vi "Get Switch Heat.vi"(8 "error in (no error)":errorcluster, 11 "Instrument.1820 in":refnum<class "Instrument.Oxford1820.lvclass">) -> (0 "error out":errorcluster, 1 "Heater On?":bool, 2 "Switch Heater Status":string, 3 "Instrument.1820 in":refnum<class "Instrument.Oxford1820.lvclass">)   [LabVIEW 2016, in "Instrument.Oxford1820.lvclass"]
uses:
  Instrument.Oxford1820.lvclass
  Typedefs/Instrument.Oxford1820.Commands-enum.ctl
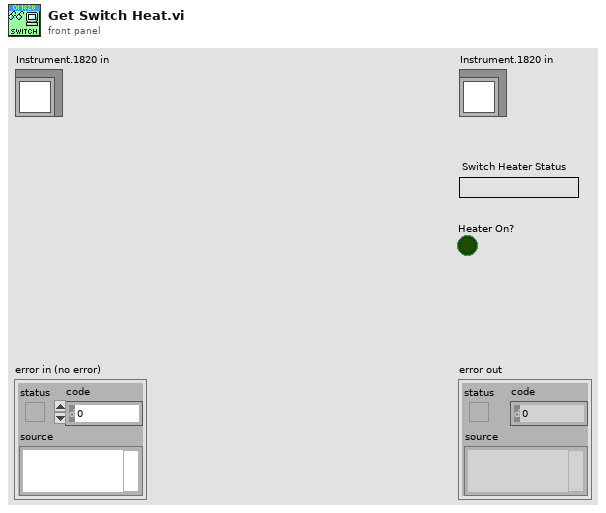
[diagram p1: front panel]
types:
  T1 = typedef "Instrument.Oxford1820.lvclass/Instrument.Oxford1820.Commands-enum.ctl" = enum16{"setAction", "setTarget", "setSwitchHeat", "setLambda", "setFillMode", "setNeedleValve", "setMagnetField", "getStatus", "getTarget", "getSwitchHeat", "getPSUField", "getMagnetField"}
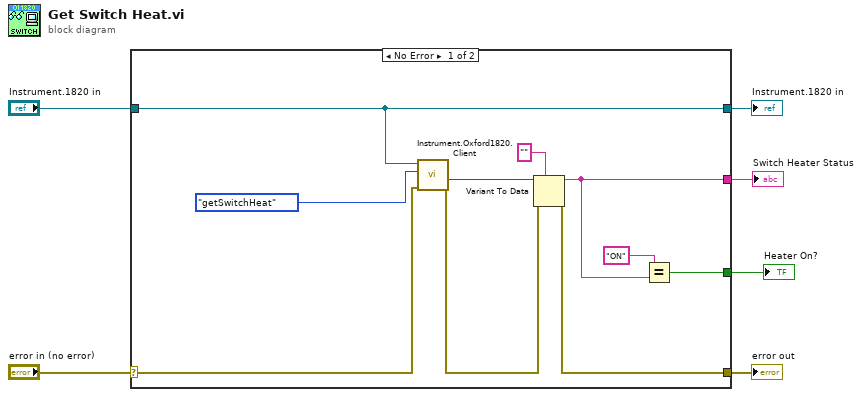
[diagram p0: block diagram]
diagram:
  n1 = case shown="No Error" "error in (no error)" {
    selector: "error in (no error)" -> [w8 w18]
    tunnel: [w14 w18] -> w5
    tunnel: [w7 w17] -> w3
    tunnel: "Instrument.1820 in" -> [w7 w17]
    tunnel: [w11 _] -> w2
    tunnel: [w10 _] -> w1
    frame No Error {
      n2 = call "Instrument.Oxford1820.Client.vi"("error in (no error)"=w8, "Commands"=Instrument.Oxford1820.Commands-enum."getSwitchHeat", "Instrument.1820 in"=w7) -> ("error out"=w15:errorcluster, "Data out"=w16:variant)  [unwired: 6 in, 1 out]
      n3 = Variant To Data(error in=w15, type="", Variant=w16) -> (data=w11:string, error out=w14:errorcluster)
      n4 = Equal?(x="ON", y=w11) -> (x = y?=w10:bool)
    }
    frame Error {
    }
  }
  "error out" <- w5
  "Instrument.1820 in" <- w3
  "Switch Heater Status" <- w2
  "Heater On?" <- w1
